vi "publish.vi"(7 "QoS":T1, 8 "error in":errorcluster, 9 "data":string, 10 "topic":string, 11 "MQTT Context in":u64) -> (0 "error out":errorcluster, 2 "send ID":i32, 3 "MQTT Context out":u64)   [LabVIEW 2013, in "MQTT.lvlib"]
uses:
  MQTT.lvlib
  QoS.ctl
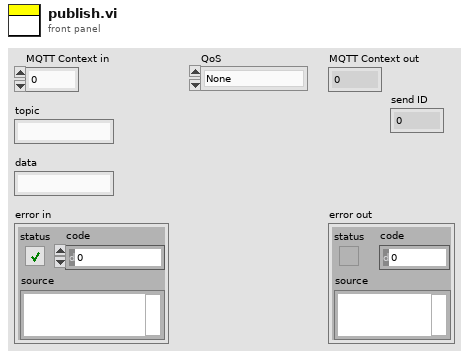
[diagram p1: front panel]
types:
  T1 = typedef "MQTT.lvlib/QoS.ctl" = enum8{"None", "At least once", "Exactly once"}
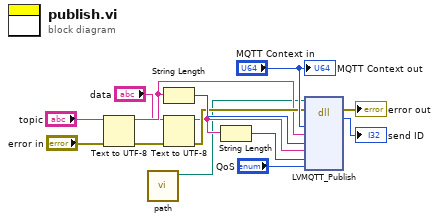
[diagram p0: block diagram]
diagram:
  n1 = Text to UTF-8(8:"error in", 11:"topic") -> (0:w7:errorcluster, 3:w4:string)
  n2 = call "path.vi"() -> ("Path"=w1:path)  [unwired: 11 in]
  n3 = String Length(string=w4) -> (length=w14:i32)
  n4 = Text to UTF-8(8:w7, 11:"data") -> (0:w6:errorcluster, 3:w2:string)
  n5 = String Length(string=w2) -> (length=w13:i32)
  n6 = dll-call lib="paho-mqtt3a.dll" fn="LVMQTT_Publish"(path in=w1, error in=w6, "lvctx"="MQTT Context in", "topic"=w4, "topiclen"=w14, "msgdata"=w2, "msglen"=w13, "qos"="QoS") -> (error out=→"error out":errorcluster, "return type"=→"send ID":i32)  [unwired: 7 in, 1 out]
  "MQTT Context out" <- "MQTT Context in"
